vi "Summarise.vi"(0 "Channel Names":string[](array[string]), 1 "Data":string[][](array[string]), 3 "Summarise All":bool) -> (5 "Summary":string[][](array[string]))   [LabVIEW 2010]
uses:
  Results_plotter_Global.vi
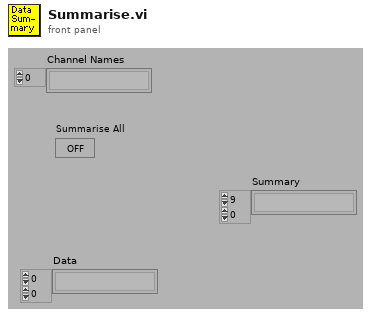
[diagram p1: front panel]
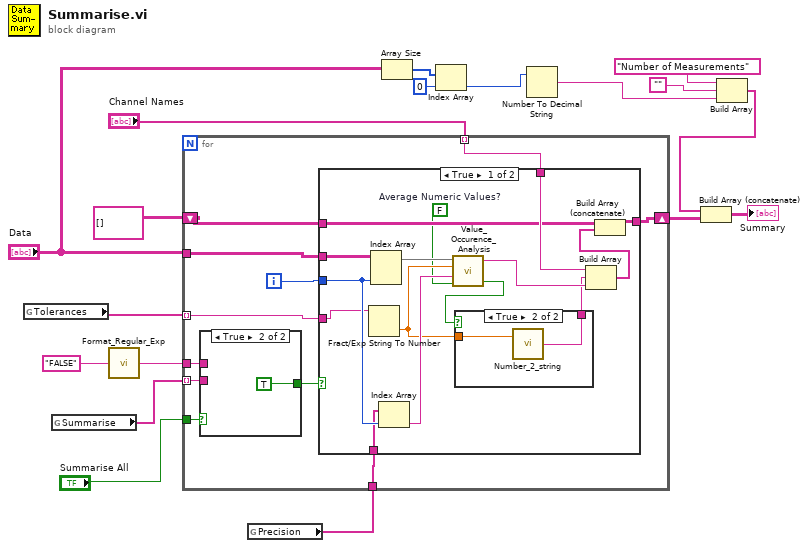
[diagram p0: block diagram]
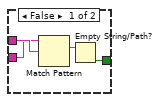
[diagram p2: hidden frame]
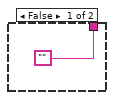
[diagram p3: hidden frame]
diagram:
  n1 = global read "Results_plotter_Global.vi" "Tolerances"() -> (w15:string[])
  n2 = global read "Results_plotter_Global.vi" "Summarise"() -> (w12:string[])
  n3 = call "Format_Regular_Exp.vi"("Regular expression"="FALSE" ("y")) -> ("Case Insensitive for html"=w13:string)
  n4 = global read "Results_plotter_Global.vi" "Precision"() -> (w16:string[])
  n5 = for {
    tunnel: "Data" -> [w29]
    tunnel: w15 -> [w26] mode=indexing
    tunnel: "Channel Names" -> [w27] mode=indexing
    shift-right: [w24] -> w2
    shift-left: string[][] [] -> [w25]
    tunnel: w16 -> [w23]
    tunnel: w13 -> [w22]
    tunnel: w12 -> [w21] mode=indexing
    tunnel: "Summarise All" -> [w20]
    i -> [w28]
    n6 = case shown="True" w20 {
      tunnel: w22 -> [w33 _]
      tunnel: w21 -> [w32 _]
      tunnel: [w30 TRUE] -> w19
      frame False {
        n7 = Match Pattern(string=w32, regular expression=w33) -> (match substring=w31:string)  [unwired: 4 out]
        n8 = Empty String/Path?(string/path=w31) -> (empty?=w30:bool)
      }
      frame True {
      }
    }
    n9 = case shown="True" w19 {
      tunnel: w29 -> [w49 _]
      tunnel: w28 -> [w40 _]
      tunnel: w27 -> [w47 _]
      tunnel: w26 -> [w37 _]
      tunnel: w25 -> [w45 w53]
      tunnel: [w44 w53] -> w24
      tunnel: w23 -> [w39 _]
      frame True {
        w35 = FALSE  # Average Numeric Values?
        n10 = Fract/Exp String To Number(string=w37) -> (number=w36:dbl)  [unwired: 4 out]
        n11 = Index Array(array=w49, index (col)=w40) -> (element=w48:string[])  [unwired: 1 in]
        n12 = Index Array(array=w39, index=w40) -> (element=w38:string)
        n13 = call "Value_Occurence_Analysis.vi"("Average Numeric Values?"=w35, "Tolerance"=w36, "Precision (3)"=w38, "String Array"=w48) -> ("Numeric Array?"=w41:bool, "Output String"=w46:string)  [unwired: 1 out]
        n14 = case shown="True" w41 {
          tunnel: w36 -> [_ w52]
          tunnel: ["" w51] -> w42
          frame False {
          }
          frame True {
            n15 = call "Number_2_string.vi"("number"=w52) -> ("String"=w51:string)  [unwired: 1 in]
          }
        }
        n16 = Build Array(w47, w42, w46) -> (w43:string[])
        n17 = Build Array (concatenate)(w45, w43) -> (w44:string[][])
      }
      frame False {
      }
    }
  }
  n18 = Array Size(array="Data") -> (size(s)=w9:i32[])
  n19 = Index Array(array=w9, index=0) -> (element=w7:i32)
  n20 = Number To Decimal String(number=w7) -> (decimal integer string=w5:string)  [unwired: 1 out]
  n21 = Build Array("Number of Measurements", "", w5) -> (w1:string[])
  n22 = Build Array (concatenate)(w1, w2) -> (→"Summary":string[][])
